vi "Filter_Evaluator.vi"(7 "Headers":string[](array[string])=["Packet Number", "Timestamp", "Source", "Destination", "Protocol", "Length", "Data"], 9 "Comparators":T1(array[cluster]), 10 "Boolean Connectors":string[](array[string])=["AND", "OR"], 11 "Prefiltered Data":string[][](array[string])=array1500x7[10500 elements]) -> (2 "Filtered Array":string[][](array[string]), 3 "Preiltered Data":string[][](array[string]))   [LabVIEW 2025, in "Table_Filtering.lvlib"]
uses:
  Table_Filtering.lvlib
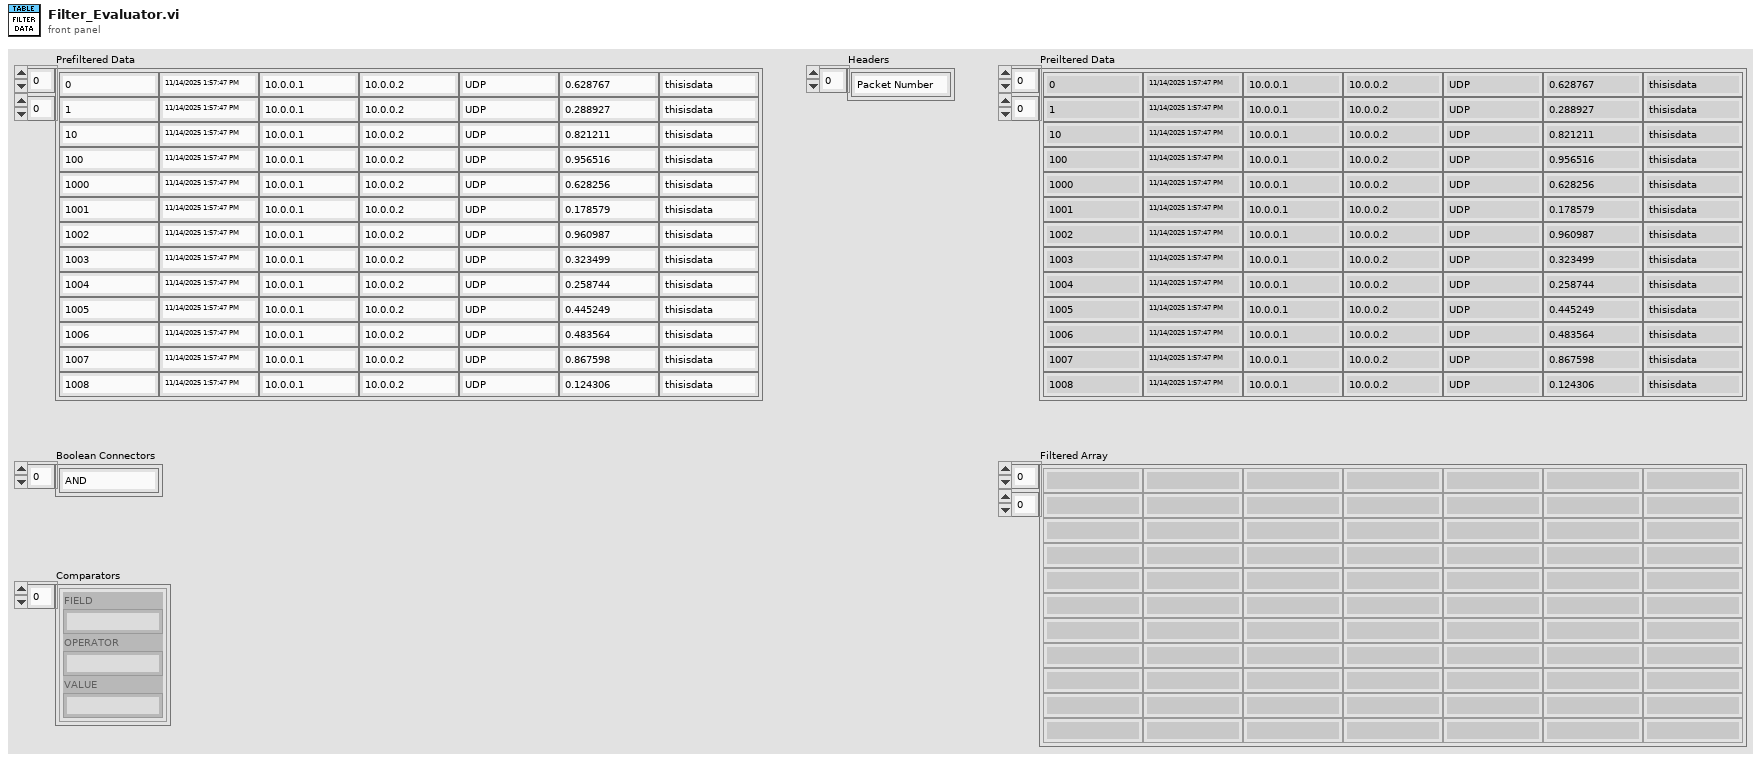
[diagram p1: front panel]
types:
  T1 = cluster{"FIELD":string, "OPERATOR":string, "VALUE":string}[]
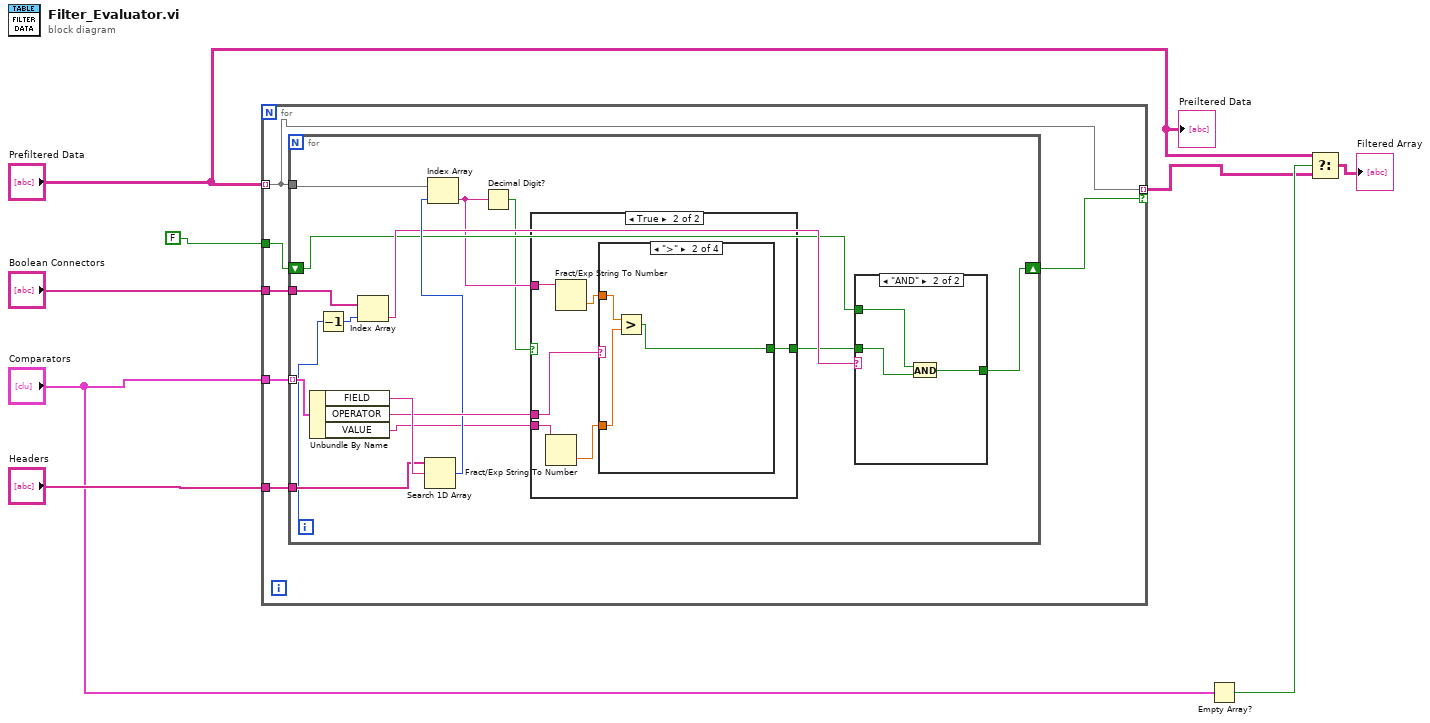
[diagram p0: block diagram]
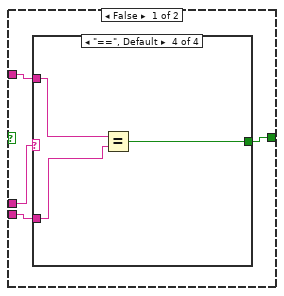
[diagram p2: hidden frame]
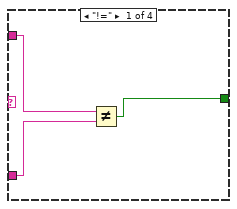
[diagram p3: hidden frame]
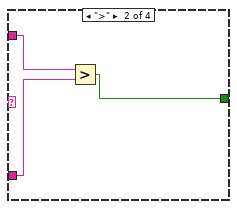
[diagram p4: hidden frame]
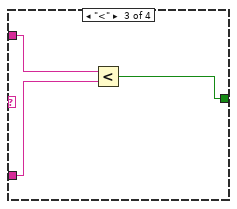
[diagram p5: hidden frame]
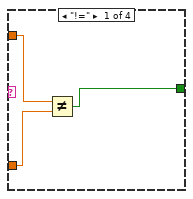
[diagram p6: hidden frame]
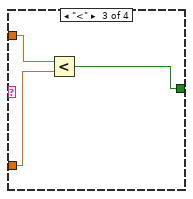
[diagram p7: hidden frame]
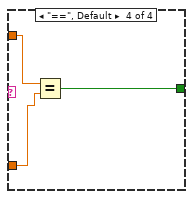
[diagram p8: hidden frame]
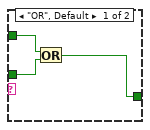
[diagram p9: hidden frame]
diagram:
  n1 = for {
    tunnel: "Headers" -> [w14]
    tunnel: "Comparators" -> [w13]
    tunnel: "Prefiltered Data" -> [w9] mode=indexing
    tunnel: FALSE -> [w12]
    tunnel: "Boolean Connectors" -> [w11]
    tunnel: [w9] -> w2 mode=indexing if=w10
    n2 = for {
      tunnel: w14 -> [w27]
      tunnel: w13 -> [w30] mode=indexing
      tunnel: w9 -> [w29]
      shift-right: [w17] -> w10
      shift-left: w12 -> [w18]
      tunnel: w11 -> [w23]
      i -> [w21]
      n3 = Unbundle By Name(w30) -> ("FIELD"=w28:string, "OPERATOR"=w26:string, "VALUE"=w24:string)
      n4 = Decrement(x=w21) -> (x-1=w22:i32)
      n5 = Index Array(array=w23, index=w22) -> (element=w20:string)
      n6 = Search 1D Array(1D array=w27, element=w28) -> (index of element=w25:i32)  [unwired: 1 in]
      n7 = Index Array(array=w29, index=w25) -> (element=w16:string)
      n8 = Decimal Digit?(1:w16) -> (0:w15:bool)
      n9 = case shown="True" w15 {
        tunnel: w26 -> [w33 w52]
        tunnel: w24 -> [w32 w49]
        tunnel: [w31 w51] -> w19
        tunnel: w16 -> [w34 w48]
        frame False {
          n10 = case shown="\"==\", Default" w33 {
            tunnel: w34 -> [w36 w40 w43 w44]
            tunnel: w32 -> [w35 w39 w42 w46]
            tunnel: [w37 w38 w41 w45] -> w31
            frame "!=" {
              n11 = Not Equal?(x=w36, y=w35) -> (x != y?=w37:bool)
            }
            frame ">" {
              n12 = Greater?(x=w40, y=w39) -> (0:w38:bool)
            }
            frame "<" {
              n13 = Less?(x=w43, y=w42) -> (x < y?=w41:bool)
            }
            frame "==", Default {
              n14 = Equal?(x=w44, y=w46) -> (x = y?=w45:bool)
            }
          }
        }
        frame True {
          n15 = Fract/Exp String To Number(string=w49) -> (number=w50:dbl)  [unwired: 3 in, 1 out]
          n16 = Fract/Exp String To Number(string=w48) -> (number=w47:dbl)  [unwired: 3 in, 1 out]
          n17 = case shown="\">\"" w52 {
            tunnel: w50 -> [w54 w58 w61 w64]
            tunnel: [w55 w57 w60 w63] -> w51
            tunnel: w47 -> [w53 w56 w59 w62]
            frame "!=" {
              n18 = Not Equal?(x=w53, y=w54) -> (x != y?=w55:bool)
            }
            frame ">" {
              n19 = Greater?(x=w56, y=w58) -> (0:w57:bool)
            }
            frame "<" {
              n20 = Less?(x=w59, y=w61) -> (x < y?=w60:bool)
            }
            frame "==", Default {
              n21 = Equal?(x=w62, y=w64) -> (x = y?=w63:bool)
            }
          }
        }
      }
      n22 = case shown="\"AND\"" w20 {
        tunnel: w19 -> [w66 w70]
        tunnel: w18 -> [w65 w69]
        tunnel: [w67 w68] -> w17
        frame "OR", Default {
          n23 = Or(x=w65, y=w66) -> (x .or. y?=w67:bool)
        }
        frame "AND" {
          n24 = And(x=w69, y=w70) -> (x .and. y?=w68:bool)
        }
      }
    }
  }
  n25 = Empty Array?(array="Comparators") -> (empty?=w4:bool)
  n26 = Select(t="Prefiltered Data", s=w4, f=w2) -> (s? t:f=→"Filtered Array":string[][])
  "Preiltered Data" <- "Prefiltered Data"
